vi "nifxpmath_GlobalTermNames.vi"() -> ()   [LabVIEW 2017]
doc: "Contains some globals shared by all XNodes in the library"
panel:
  in  "DNL_TERM IDS":string[](array[string])=["TERM_OVFL", "TERM_HS_ND", "TERM_HS_DR", "TERM_HS_RFD", "TERM_HS_RFO"]
  in  "TERM NAMES":string[](array[string])=["operation overflow", "input valid", "output valid", "ready for input", "ready for output (T)"]
  in  "DNL_ENGLISH NAMES":string[](array[string])=["operation overflow", "input valid", "output valid", "ready for input", "ready for output (T)"]
  # "This global VI must be marked for localization, and contains terminal English names, localized names, and IDs\nfor the overflow and handshaking terminals.\nAll controls have captions, since we only want to localize the data, not the labels."
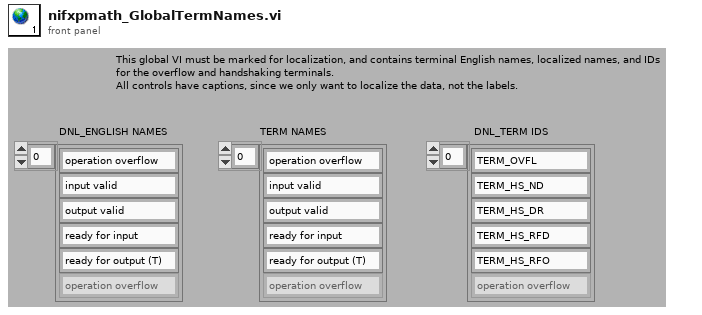
[diagram p1: front panel]
diagram:
